vi "json Parse Double - string path.vi"(8 "error in (no error)":errorcluster, 9 "default":dbl, 10 "path":string, 11 "JSON Document in":refnum<class "JSON Document.lvclass">) -> (0 "error out":errorcluster, 1 "defaulted?":bool, 2 "value":dbl, 3 "JSON Document out":refnum<class "JSON Document.lvclass">)   [LabVIEW 2015, in "JSON Document.lvclass"]
uses:
  JSON Document.lvclass
  JSON Document.lvclass/JSON Document.ctl
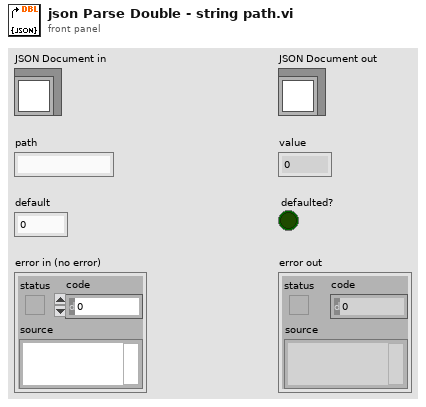
[diagram p1: front panel]
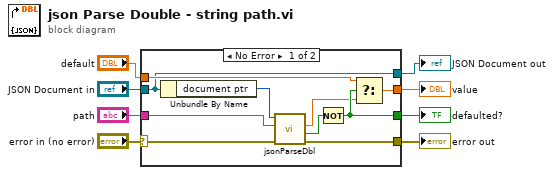
[diagram p0: block diagram]
diagram:
  n1 = case shown="No Error" "error in (no error)" {
    selector: "error in (no error)" -> [w18 w21]
    tunnel: [w15 w21] -> w5
    tunnel: [w14 w20] -> w2
    tunnel: "JSON Document in" -> [w14 w20]
    tunnel: "default" -> [w16 w19]
    tunnel: "path" -> [w12 _]
    tunnel: [w17 w19] -> w4
    tunnel: [w13 _] -> w3
    frame No Error {
      n2 = Unbundle By Name(w14) -> ("document ptr"=w11:i64)
      n3 = call "jsonParseDbl.vi"("error in (no error)"=w18, "path"=w12, "d in"=w11) -> ("error out"=w15:errorcluster, "success?"=w10:bool, "value"=w9:dbl)  [unwired: 5 in, 1 out]
      n4 = Not(x=w10) -> (.not. x?=w13:bool)
      n5 = Select(t=w16, s=w13, f=w9) -> (s? t:f=w17:dbl)
    }
    frame Error {
    }
  }
  "error out" <- w5
  "JSON Document out" <- w2
  "value" <- w4
  "defaulted?" <- w3
